vi "Global 2.vi"() -> ()   [LabVIEW 2015]
panel:
  out "Cam Y Pos":dbl
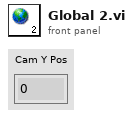
[diagram p1: front panel]
diagram:
